vi "Deallocate.vi"(8 "error in (no error)":errorcluster, 11 "Pointer":refnum<class "Pointer.lvclass">) -> (0 "error out":errorcluster, 3 "Pointer type":refnum<class "Pointer.lvclass">)   [LabVIEW 2027, in "Memory Manager.lvlib" / "Pointer.lvclass"]
doc: "Deallocates the block of memory specified by <b>Pointer</b>."
uses:
  Pointer.lvclass
  Zone.vi
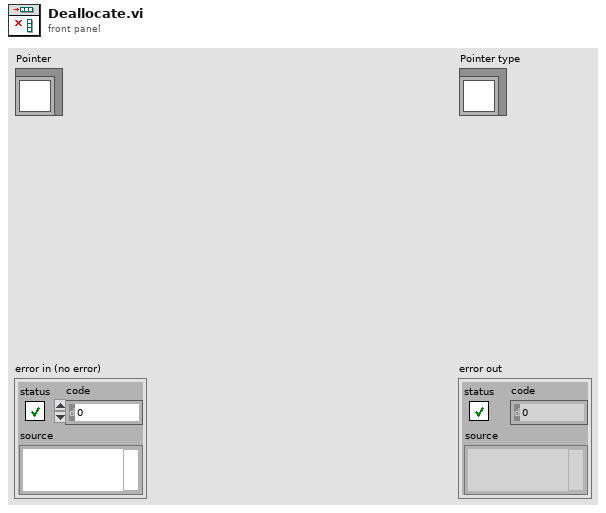
[diagram p1: front panel]
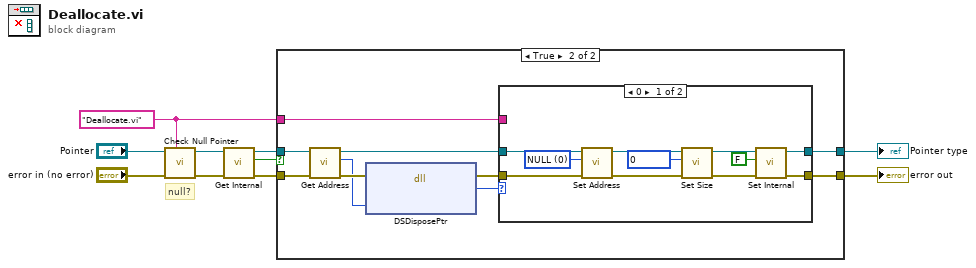
[diagram p0: block diagram]
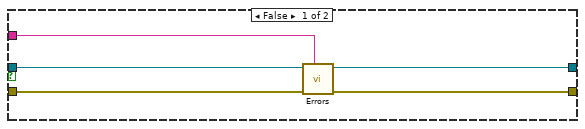
[diagram p2: hidden frame]
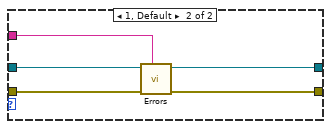
[diagram p3: hidden frame]
diagram:
  w1 = "Deallocate.vi" ("source vi name")
  # "null?"
  n1 = call "Check Null Pointer.vi"("source vi name"=w1, "error in (no error)"="error in (no error)", "Pointer in"="Pointer") -> ("error out"=w2:errorcluster, "Pointer out"=w3:refnum<class "Pointer.lvclass">)  [unwired: 7 in]
  n2 = call "Get Internal.vi"("Pointer in"=w3) -> ("internal"=w6:bool, "Pointer out"=w7:refnum<class "Pointer.lvclass">)  [unwired: 9 in]
  n3 = case shown="True" w6 {
    tunnel: [w12 w23] -> w9
    tunnel: [w11 w22] -> w8
    tunnel: w2 -> [w13 w21]
    tunnel: w7 -> [w14 w16]
    tunnel: w1 -> [w10 w15]
    frame False {
      n4 = call-poly "Errors.vi"("error source vi name"=w10, "error in (no error)"=w13, "Pointer in"=w14) -> ("error out"=w11:errorcluster, "Pointer out"=w12:refnum<class "Pointer.lvclass">)  [unwired: 7 in]
    }
    frame True {
      n5 = call "Get Address.vi"("Pointer in"=w16) -> ("address"=w17:u64, "Pointer out"=w18:refnum<class "Pointer.lvclass">)  [unwired: 9 in]
      n6 = dll-call lib="LabVIEW" fn="DSDisposePtr"(error in=w21, "pointer"=w17) -> (error out=w20:errorcluster, "return"=w19:i32)  [unwired: 3 in, 1 out]
      n7 = case shown="0" w19 {
        tunnel: w20 -> [w27 w36]
        tunnel: [w27 w35] -> w22
        tunnel: [w25 w34] -> w23
        tunnel: w18 -> [w31 w33]
        tunnel: w15 -> [_ w32]
        frame 0 {
          w28 = u64 0 items=["NULL"] ("Null")
          n8 = call "Set Address.vi"("address"=w28, "Pointer in"=w31) -> ("Pointer out"=w30:refnum<class "Pointer.lvclass">)  [unwired: 9 in]
          n9 = call "Set Size.vi"("size"=u64 0, "Pointer in"=w30) -> ("Pointer out"=w26:refnum<class "Pointer.lvclass">)  [unwired: 9 in]
          n10 = call "Set Internal.vi"("internal"=FALSE, "Pointer in"=w26) -> ("Pointer out"=w25:refnum<class "Pointer.lvclass">)  [unwired: 9 in]
        }
        frame 1, Default {
          n11 = call-poly "Errors.vi"("error source vi name"=w32, "error in (no error)"=w36, "Pointer in"=w33) -> ("error out"=w35:errorcluster, "Pointer out"=w34:refnum<class "Pointer.lvclass">)  [unwired: 7 in]
        }
      }
    }
  }
  "error out" <- w8
  "Pointer type" <- w9
